vi "p3.vi"() -> ()   [LabVIEW 2015]
panel:
  in  "milliseconds to wait":u32=210
  in  "Stop Button":bool
  out "Numeric Indicator 2":u32
  out "Numeric Indicator":u32
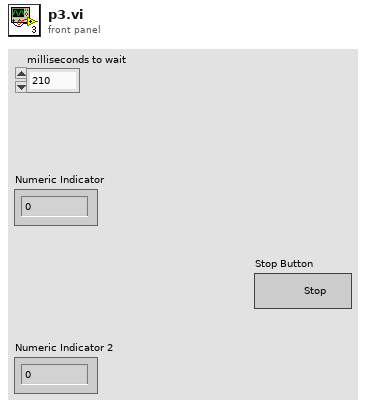
[diagram p1: front panel]
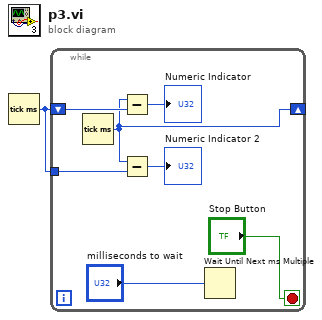
[diagram p0: block diagram]
diagram:
  n1 = Tick Count (ms)() -> (millisecond timer value=w1:u32)
  n2 = while {
    shift-right: [w4] -> _
    shift-left: w1 -> [w5]
    tunnel: w1 -> [w3]
    stop <- "Stop Button" stop-if-true
    n3 = Tick Count (ms)() -> (millisecond timer value=w4:u32)
    n4 = Subtract(x=w4, y=w5) -> (x-y=→"Numeric Indicator":u32)
    n5 = Subtract(x=w4, y=w3) -> (x-y=→"Numeric Indicator 2":u32)
    n6 = Wait Until Next ms Multiple(millisecond multiple="milliseconds to wait") -> ()  [unwired: 1 out]
  }
